vi "Autonomous Init.vi"   [LabVIEW 2017]
uses:
  Robot Global Data.vi
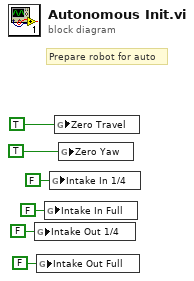
[diagram p0: block diagram]
diagram:
  # "Prepare robot for auto"
  n1 = global write "Robot Global Data.vi" "Intake Out 1/4"(FALSE ("Intake Out 1/4")) -> ()
  n2 = global write "Robot Global Data.vi" "Intake Out Full"(FALSE ("Intake Out Full")) -> ()
  n3 = global write "Robot Global Data.vi" "Intake In Full"(FALSE ("Intake In Full")) -> ()
  n4 = global write "Robot Global Data.vi" "Intake In 1/4"(FALSE ("Intake In 1/4")) -> ()
  n5 = global write "Robot Global Data.vi" "Zero Travel"(TRUE) -> ()
  n6 = global write "Robot Global Data.vi" "Zero Yaw"(TRUE) -> ()
